vi "FTW-CodeGen-XNodeUpdateState.vi"(0 "XRef":refnum<vi>, 5 "Version":T1, 11 "error in":errorcluster) -> (6 "Reply":string[](array[string]))   [LabVIEW 2014]
uses:
  FTW-CodeGen-XNodeReplyType.ctl
panel:
  # "Inputs"
  # "Outputs"
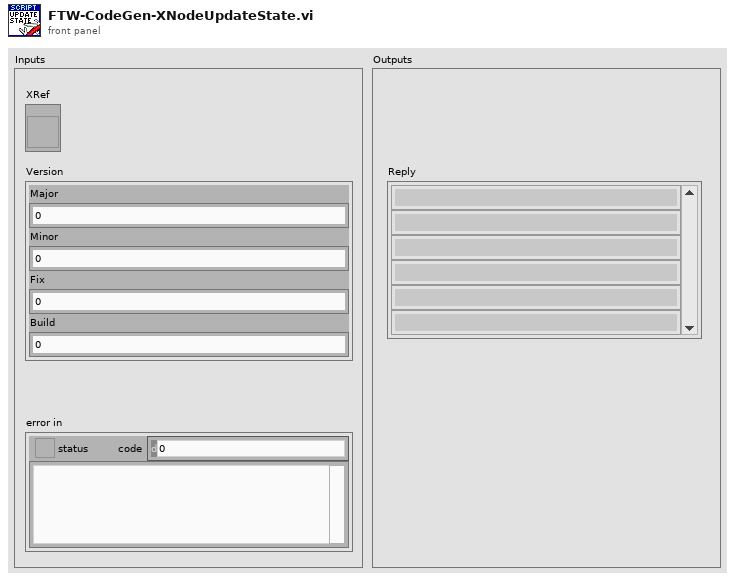
[diagram p1: front panel]
types:
  T1 = cluster{"Major":u16, "Minor":u16, "Fix":u16, "Build":u16}
  T2 = typedef "FTW-CodeGen-XNodeReplyType.ctl" = enum16{"Update State", "AdaptToInputs", "CosmeticUpdate", "No Reply"}
  T3 = cluster{"Major":bool, "Minor":bool, "Fix":bool, "Build":bool}
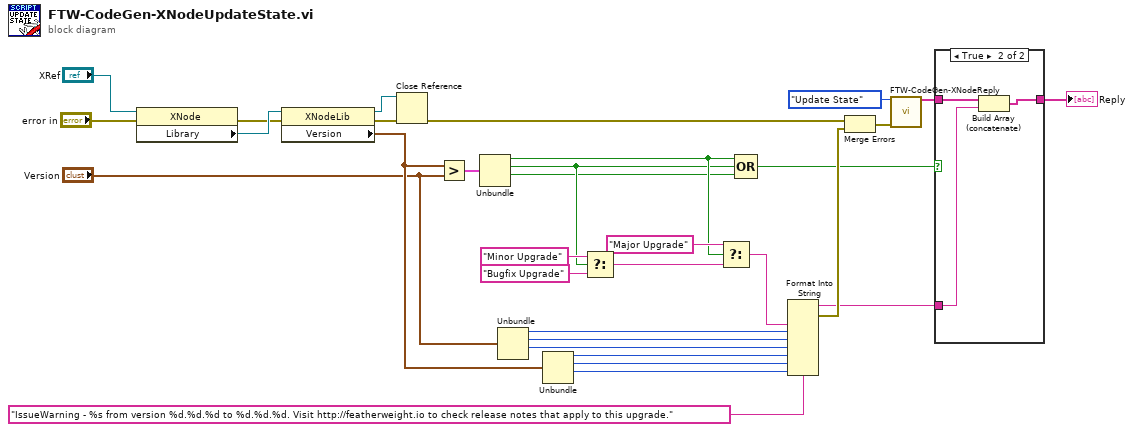
[diagram p0: block diagram]
diagram:
  n1 = property class="XNode"(reference="XRef", error in="error in") -> (error out=w17:errorcluster, "Library"=w30:refnum<vi>)  [unwired: 1 out]
  n2 = property class="XNodeLib"(reference=w30, error in=w17) -> (reference out=w4:refnum<vi>, error out=w3:errorcluster, "Version"=w6:T1)
  n3 = Close Reference(reference=w4, error in (no error)=w3) -> (error out=w2:errorcluster)
  n4 = Greater?(x=w6, y="Version") -> (0:w29:T3)
  n5 = Unbundle(w29) -> ("Major"=w13:bool, "Minor"=w12:bool, "Fix"=w11:bool)  [unwired: 1 out]
  n6 = Unbundle("Version") -> ("Major"=w28:u16, "Minor"=w27:u16, "Fix"=w26:u16)  [unwired: 1 out]
  n7 = Unbundle(w6) -> ("Major"=w25:u16, "Minor"=w24:u16, "Fix"=w23:u16)  [unwired: 1 out]
  n8 = Select(t="Minor Upgrade", s=w12, f="Bugfix Upgrade") -> (s? t:f=w19:string)
  n9 = Select(t="Major Upgrade", s=w13, f=w19) -> (s? t:f=w18:string)
  n10 = Compound Arithmetic op=OR(w13, w12, w11) -> (w7:bool)
  n11 = Format Into String(format string="IssueWarning - %s from version %d.%d.%d to %d.%d.%d. Visit http://featherweight.io to check release notes that apply to this upgrade.", w18, w28, w27, w26, w25, w24, w23) -> (resulting string=w8:string, error out=w16:errorcluster)  [unwired: 2 in]
  n12 = Merge Errors(w2, w16) -> (w15:errorcluster)
  n13 = call "FTW-CodeGen-XNodeReply.vi"("XNode Reply Type"=FTW-CodeGen-XNodeReplyType."Update State", "error in"=w15) -> ("Reply"=w10:string[])  [unwired: 13 in]
  n14 = case shown="True" w7 {
    tunnel: w10 -> [w33 w36]
    tunnel: [w33 w35] -> w9
    tunnel: w8 -> [_ w34]
    frame False {
    }
    frame True {
      n15 = Build Array (concatenate)(w36, w34) -> (w35:string[])
    }
  }
  "Reply" <- w9
